vi "Read Value.vi"(8 "error in (no error)":errorcluster, 11 "Update Tag Config in":refnum<class "Update Tag Config.lvclass">) -> (0 "error out":errorcluster, 2 "Value":variant, 3 "Update Tag Config out":refnum<class "Update Tag Config.lvclass">)   [LabVIEW 2015, in "Update Tag Config.lvclass"]
uses:
  Update Tag Config.lvclass
  Update Tag Config.lvclass/Update Tag Config.ctl
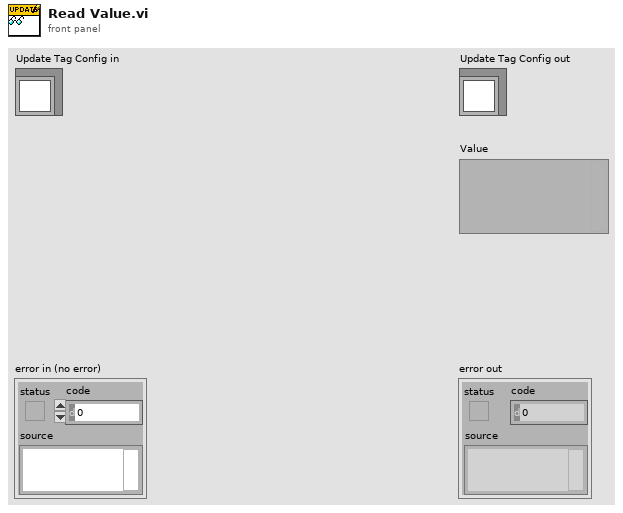
[diagram p1: front panel]
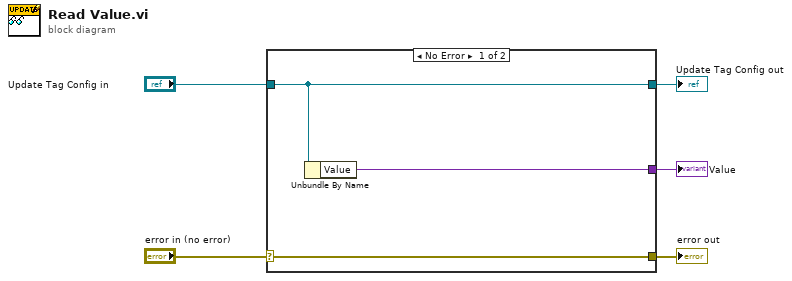
[diagram p0: block diagram]
diagram:
  n1 = case shown="No Error" "error in (no error)" {
    selector: "error in (no error)" -> [w8 w9]
    tunnel: [w8 w9] -> w4
    tunnel: [w7 w10] -> w2
    tunnel: "Update Tag Config in" -> [w7 w10]
    tunnel: [w6 _] -> w1
    frame No Error {
      n2 = Unbundle By Name(w7) -> ("Value"=w6:variant)
    }
    frame Error {
    }
  }
  "error out" <- w4
  "Update Tag Config out" <- w2
  "Value" <- w1
